vi "Reserve Intake_wrapper.vi"() -> ()   [LabVIEW 2019]
uses:
  <vilib>/Rock Robotics/WPI/Framework/Completion Status.ctl
  <vilib>/Rock Robotics/WPI/Framework/Completion Notifier.ctl
  <vilib>/Rock Robotics/WPI/Framework/Command Status Info.ctl
panel:
  out "Command Info 2":T1
  in  "Command Name":string
  in  "Command Info":T1
  in  "Description":string="Reserve"
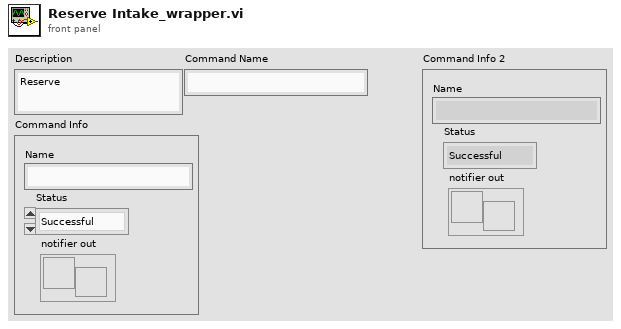
[diagram p1: front panel]
types:
  T1 = typedef "Command Status Info.ctl" = cluster{"Name":string, "Status":T2, "notifier out":T3}
  T2 = typedef "Completion Status.ctl" = enum16{"Successful", "Aborted", "Incomplete"}
  T3 = typedef "Completion Notifier.ctl" = refnum<notifier>
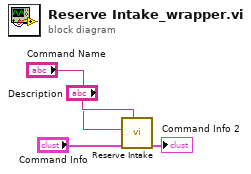
[diagram p0: block diagram]
diagram:
  n1 = call "Reserve Intake.vi"("Description"="Description", "Command Info"="Command Info", "Command Name"="Command Name") -> ("Command Info"=→"Command Info 2":T1)  [unwired: 8 in]
